vi "Init.vi"(9 "Relation":T1, 10 "Self Attributes":refnum<class "Attributes.lvclass">) -> (2 "Teller":refnum<class "Teller.lvclass">)   [LabVIEW 2025, in "jettl.lvlib" / "Teller.lvlib"]
uses:
  Teller.lvlib
  Teller/Teller.lvclass
  Attributes/Attributes/Attributes.lvclass
  Relation.ctl
  Base Teller/Base Teller.lvclass
  jettl.lvlib
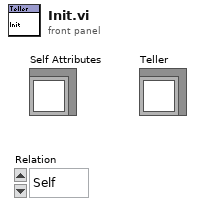
[diagram p1: front panel]
types:
  T1 = typedef "jettl.lvlib/Relation.ctl" = enum16{"Self", "Parent", "Child"}
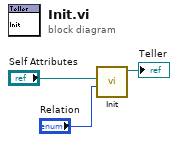
[diagram p0: block diagram]
diagram:
  n1 = call "Init.vi"("Relation"="Relation", "Self Attributes"="Self Attributes") -> ("Base Teller out"=→"Teller":refnum<class "Base Teller.lvclass">)  [unwired: 9 in]
